vi "Solartron 1260 freq scan with averaging.vi"(0 "VISA resource name":refnum<visa-resource-name>="GPIB2::4::INSTR", 11 "error in (no error)":errorcluster) -> ()   [LabVIEW 2014]
doc: "This VI configures and reads back a single measurement. \n\nNote:\nYou might need to extend the timeout set in the Wait Conditions subVI."
uses:
  <vilib>/Utility/file.llb/Write To Spreadsheet File (string).vi
  <instrlib>/Solartron 1260/Solartron 1260.lvlib
panel:
  out "scan time (hrs)":dbl
  out "scan time (min)":dbl
  in  "stop":bool
  out "Step size (Hz)":dbl
  out "XY Graph 3":cluster{dbl[], dbl[]}[](graph)
  in  "Frequency options":T1={"End freq (Hz)"=0.0, "Start freq (Hz)"=0.0, "# of steps"=0.0, "# of steps to average"=3.0} {"Start freq (Hz)" format="%#_8f"; "End freq (Hz)" format="%#_8f"}
  in  "Variable, result source, citcuit":T2={"Variable (0:Frequency)"=enum."Frequency", "Result Source(0:Z1 = V1/I)"=enum."Z1 = V1/I", "Circuit (3:Parallel C, R)"=enum."Serial L, R", "Result Type(0: [Z, Theta] for: Z1 or Z2)"=enum."[Z, Theta]       for: Z1 or Z2", "DC Bias (V)"=0.0, "Amplitude (V)"=1.0} {"Amplitude (V)" min=0.0 max=3.0 format="%^.3e"; "DC Bias (V)" min=-42.0 max=42.0 format="%^.3e"}
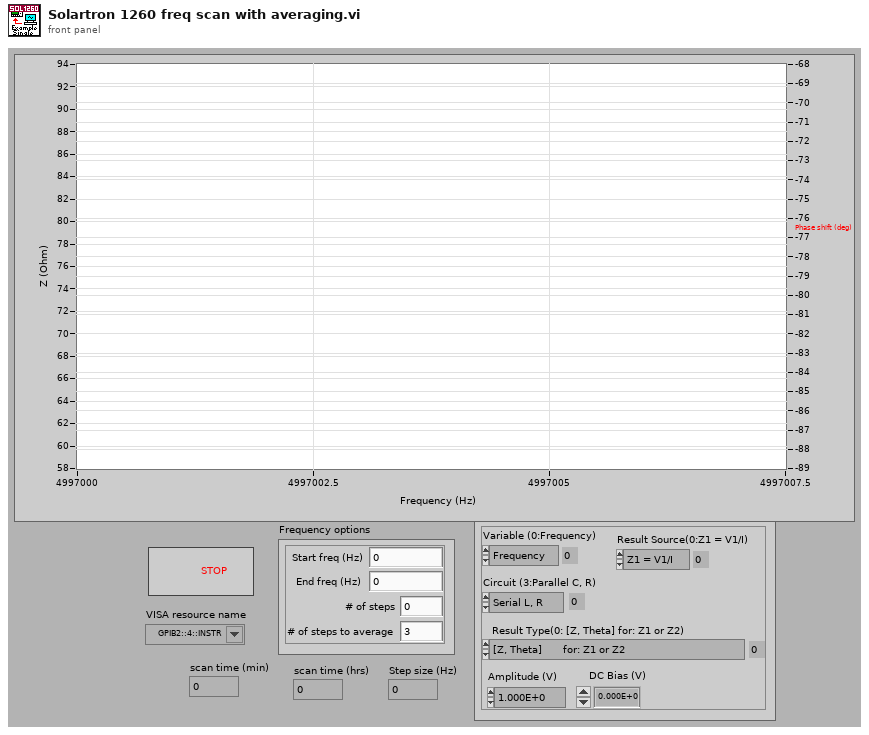
[diagram p1: front panel]
types:
  T1 = cluster{"End freq (Hz)":dbl, "Start freq (Hz)":dbl, "# of steps":dbl, "# of steps to average":dbl}
  T2 = cluster{"Variable (0:Frequency)":enum16{"Frequency", "Amplitude", "Baise"}, "Result Source(0:Z1 = V1/I)":enum16{"Z1 = V1/I", "Y1 = I/V1", "Z2 = V2/I", "Y2 = I/V2", "Function (  )", "V1", "V2", "V1/V2", "V2/V1", " I"}, "Circuit (3:Parallel C, R)":enum16{"Serial L, R", "Serial C, R", "Parallel L, R", "Parallel C, R", "Auto"}, "Result Type(0: [Z, Theta] for: Z1 or Z2)":enum16{"[Z, Theta]       for: Z1 or Z2", "[Y, Theta]       for: Y1 or Y2", "[r, Theta]        for: Fnc( ), V1, V2, V1/V2, V2/V1 or I", "[r(dB), Theta]  for: Fnc( ), V1, V2, V1/V2 or V2/V1", "[r, t]                 for: Fnc( ), V1, V2, V1/V2 or V2/V1", "[r (dB), t]          for: Fnc( ), V1, V2, V1/V2 or V2/V1", "[L(or C), R]      for: Z1, Y1, Z2, Y2 or Fnc( )", "[L(or C), Q]      for: Z1, Y1, Z2, Y2 or Fnc( )", "[L(or C), D]      for: Z1, Y1, Z2, Y2 or Fnc( ) ", "[R, X]              for: Z1 or Z2", "[G, B]              for: Y1 or Y2", "[a, b]               for: Fnc( ), V1, V2, V1/V2, V2/V1 or I"}, "DC Bias (V)":dbl, "Amplitude (V)":dbl}
  T3 = enum16{"Off", "All", "Fail", "Pass", "Dump", "Dump all", "Plotter"}
  T4 = enum16{"Z1 = V1/I", "Y1 = I/V1", "Z2 = V2/I", "Y2 = I/V2", "Function (  )", "V1", "V2", "V1/V2", "V2/V1", " I"}
  T5 = enum16{"Serial L, R", "Serial C, R", "Parallel L, R", "Parallel C, R", "Auto"}
  T6 = enum16{"[Z, Theta]       for: Z1 or Z2", "[Y, Theta]       for: Y1 or Y2", "[r, Theta]        for: Fnc( ), V1, V2, V1/V2, V2/V1 or I", "[r(dB), Theta]  for: Fnc( ), V1, V2, V1/V2 or V2/V1", "[r, t]                 for: Fnc( ), V1, V2, V1/V2 or V2/V1", "[r (dB), t]          for: Fnc( ), V1, V2, V1/V2 or V2/V1", "[L(or C), R]      for: Z1, Y1, Z2, Y2 or Fnc( )", "[L(or C), Q]      for: Z1, Y1, Z2, Y2 or Fnc( )", "[L(or C), D]      for: Z1, Y1, Z2, Y2 or Fnc( ) ", "[R, X]              for: Z1 or Z2", "[G, B]              for: Y1 or Y2", "[a, b]               for: Fnc( ), V1, V2, V1/V2, V2/V1 or I"}
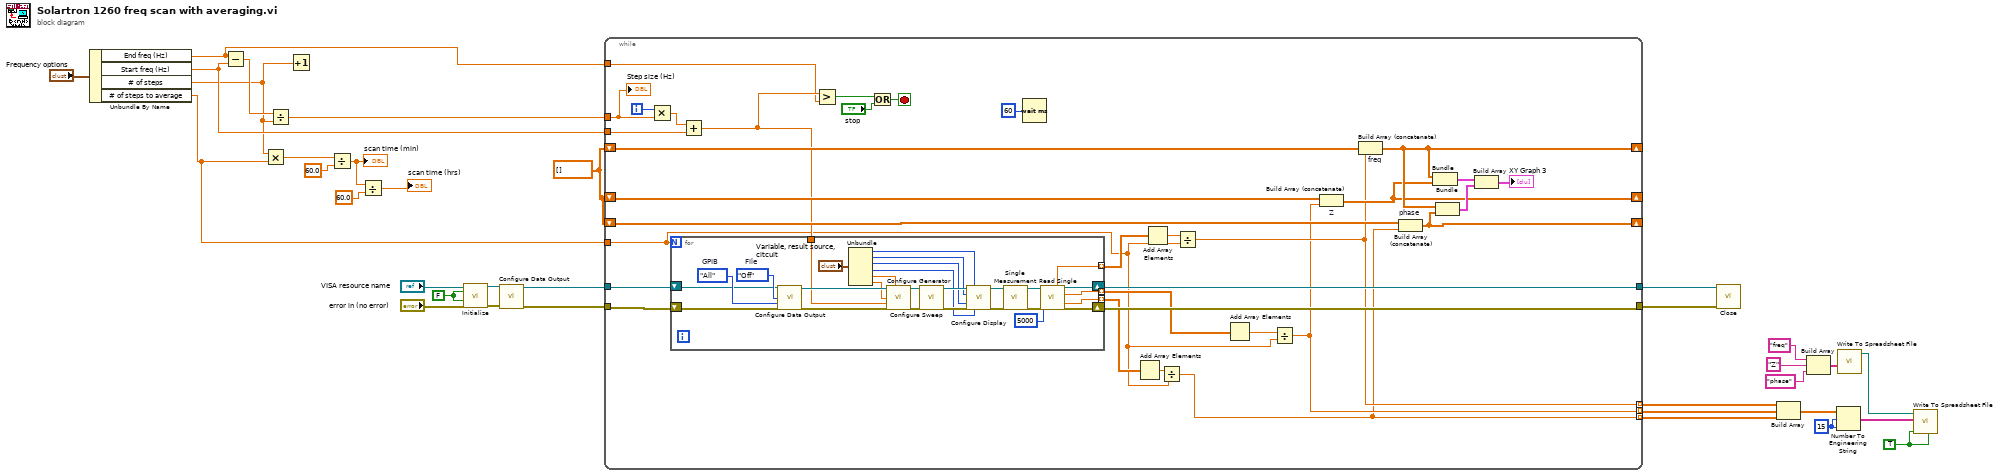
[diagram p0: block diagram]
diagram:
  w8 = TRUE ("append to file? (new file:F)")
  w16 = i16 15 ("precision (6)")
  w21 = dbl[] []
  w31 = FALSE ("ID Query (T: Check)")
  n1 = Unbundle By Name("Frequency options") -> ("End freq (Hz)"=w9:dbl, "Start freq (Hz)"=w23:dbl, "# of steps"=w3:dbl, "# of steps to average"=w1:dbl)
  n2 = Subtract(x=w9, y=w23) -> (x-y=w34:dbl)
  n3 = Multiply(x=w3, y=w1) -> (x*y=w2:dbl)
  n4 = Divide(x=w34, y=w3) -> (x/y=w22:dbl)
  n5 = Increment(x=w3) -> ()  [unwired: 1 out]
  n6 = Divide(x=w2, y=60.0) -> (x/y=w5:dbl)
  "scan time (min)" <- w5
  n7 = Divide(x=w5, y=60.0) -> (x/y=→"scan time (hrs)":dbl)
  n8 = call <instrlib>:"Initialize.vi"("VISA resource name"="VISA resource name", "ID Query (T: Check)"=w31, "Reset (T: Reset)"=w31, "error in (no error)"="error in (no error)") -> ("VISA resource name out"=w27:refnum<visa-resource-name>, "error out"=w28:errorcluster)  [unwired: 10 in]
  n9 = call <instrlib>:"Configure Data Output.vi"("VISA resource name"=w27, "error in (no error)"=w28) -> ("VISA resource name out"=w26:refnum<visa-resource-name>, "error out"=w25:errorcluster)  [unwired: 12 in]
  n10 = while {
    tunnel: [w61] -> w33
    tunnel: [w60] -> w32
    tunnel: w26 -> [w63]
    tunnel: w25 -> [w62]
    tunnel: w23 -> [w64]
    shift-right: [w51] -> _
    shift-left: w21 -> [w59]
    shift-right: [w50] -> _
    shift-left: w21 -> [w58]
    tunnel: w22 -> [w57]
    shift-right: [w53] -> _
    shift-left: w21 -> [w54]
    tunnel: [w40] -> w20 mode=indexing
    tunnel: [w36] -> w19 mode=indexing
    tunnel: [w35] -> w18 mode=indexing
    tunnel: w9 -> [w46]
    tunnel: w1 -> [w39]
    i -> [w66]
    stop <- w49 stop-if-true
    n11 = Multiply(x=w66, y=w57) -> (x*y=w65:dbl)
    n12 = Add(x=w65, y=w64) -> (x+y=w47:dbl)
    n13 = for {
      N: w39 -> [_]
      tunnel: [w73] -> w44 mode=indexing
      tunnel: [w72] -> w43 mode=indexing
      tunnel: [w71] -> w42 mode=indexing
      tunnel: w47 -> [w70]
      shift-right: [w79] -> w60
      shift-left: w63 -> [w82]
      shift-right: [w80] -> w61
      shift-left: w62 -> [w81]
      w84 = T3."All"  # GPIB
      w85 = enum16{"Off", "All", "Fail", "Pass"}."Off"  # File
      n14 = call <instrlib>:"Configure Data Output.vi"("VISA resource name"=w82, "File (1:All)"=w85, "GPIB (1:All)"=w84, "error in (no error)"=w81) -> ("VISA resource name out"=w94:refnum<visa-resource-name>, "error out"=w95:errorcluster)  [unwired: 10 in]
      n15 = Unbundle("Variable, result source, citcuit") -> ("Variable (0:Frequency)"=w77:enum16{"Frequency", "Amplitude", "Baise"}, "Result Source(0:Z1 = V1/I)"=w75:T4, "Circuit (3:Parallel C, R)"=w76:T5, "Result Type(0: [Z, Theta] for: Z1 or Z2)"=w74:T6, "DC Bias (V)"=w69:dbl, "Amplitude (V)"=w68:dbl)
      n16 = call <instrlib>:"Configure Generator.vi"("VISA resource name"=w94, "Voltage Bias(0.0 V)"=w69, "Voltage Amplitude(1.0 V)"=w68, "Frequency(1.0 Hz)"=w70, "error in (no error)"=w95) -> ("VISA resource name out"=w93:refnum<visa-resource-name>, "error out"=w92:errorcluster)  [unwired: 9 in]
      n17 = call <instrlib>:"Configure Sweep.vi"("VISA resource name"=w93, "error in (no error)"=w92) -> ("VISA resource name out"=w90:refnum<visa-resource-name>, "error out"=w91:errorcluster)  [unwired: 12 in]
      n18 = call <instrlib>:"Configure Display.vi"("VISA resource name"=w90, "Variable (0:Frequency)"=w77, "Result Source(0:Z1 = V1/I)"=w75, "Circuit (3:Parallel C, R)"=w76, "error in (no error)"=w91, "Result Type(0: [Z, Theta] for: Z1 or Z2)"=w74) -> ("VISA resource name out"=w89:refnum<visa-resource-name>, "error out"=w88:errorcluster)  [unwired: 8 in]
      n19 = call <instrlib>:"Single Measurement.vi"("VISA resource name"=w89, "error in (no error)"=w88) -> ("VISA resource name out"=w86:refnum<visa-resource-name>, "error out"=w87:errorcluster)  [unwired: 12 in]
      n20 = call <instrlib>:"Read Single.vi"("VISA resource name"=w86, "timeout ms (5000)"=u32 5000, "error in (no error)"=w87) -> ("Variable"=w73:dbl, "VISA resource name out"=w79:refnum<visa-resource-name>, "Parameter 1"=w72:dbl, "Parameter2"=w71:dbl, "error out"=w80:errorcluster)  [unwired: 6 in, 2 out]
    }
    n21 = Greater?(x=w47, y=w46) -> (0:w45:bool)
    n22 = Or(x=w45, y="stop") -> (x .or. y?=w49:bool)
    n23 = Wait (ms)(milliseconds to wait=u32 60) -> ()  [unwired: 1 out]
    n24 = Add Array Elements(numeric array=w42) -> (sum=w38:dbl)
    n25 = Add Array Elements(numeric array=w44) -> (sum=w41:dbl)
    n26 = Divide(x=w38, y=w39) -> (x/y=w35:dbl)
    n27 = Divide(x=w41, y=w39) -> (x/y=w40:dbl)
    n28 = Add Array Elements(numeric array=w43) -> (sum=w37:dbl)
    n29 = Divide(x=w37, y=w39) -> (x/y=w36:dbl)
    n30 = Build Array (concatenate) "Z"(w58, w36) -> (w50:dbl[])
    n31 = Build Array (concatenate) "freq"(w59, w40) -> (w51:dbl[])
    n32 = Build Array (concatenate) "phase"(w54, w35) -> (w53:dbl[])
    n33 = Bundle(w51, w50) -> (w56:cluster{dbl[], dbl[]})  [unwired: 1 in]
    n34 = Bundle(w51, w53) -> (w55:cluster{dbl[], dbl[]})  [unwired: 1 in]
    n35 = Build Array(w56, w55) -> (→"XY Graph 3":cluster{dbl[], dbl[]}[])
    "Step size (Hz)" <- w57
  }
  n36 = call <instrlib>:"Close.vi"("VISA resource name"=w32, "error in (no error)"=w33) -> ()  [unwired: 13 in, 1 out]
  n37 = Build Array(w20, w19, w18) -> (w17:dbl[][])
  n38 = Build Array("freq", "Z", "phase") -> (w13:string[])
  n39 = Number To Engineering String(2:w16, 3:w16, 4:w17) -> (0:w15:string[][])  [unwired: 1 in]
  n40 = call-poly <vilib>:"Write To Spreadsheet File.vi"("1D data"=w13) -> ("new file path (Not A Path if cancelled)"=w14:path)  [unwired: 7 in]
  n41 = call-poly <vilib>:"Write To Spreadsheet File.vi"("transpose? (no:F)"=w8, "append to file? (new file:F)"=w8, "2D data"=w15, "file path (dialog if empty)"=w14) -> ()  [unwired: 4 in, 1 out]
